vi "ST5 Check Errors.vi"(8 "error in (no error)":errorcluster, 10 "Scan failed":bool, 11 "Read=0":bool) -> (0 "error out":errorcluster)   [LabVIEW 2019]
uses:
  <vilib>/Utility/error.llb/DialogType.ctl
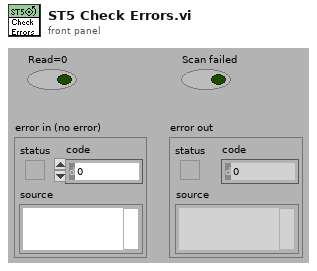
[diagram p1: front panel]
types:
  T1 = typedef "DialogType.ctl" = u16
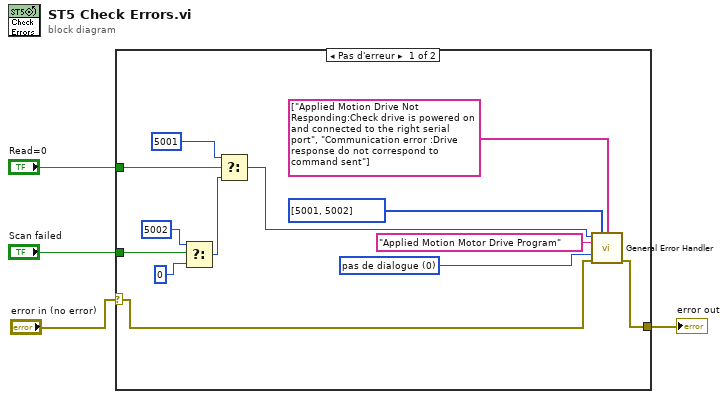
[diagram p0: block diagram]
diagram:
  n1 = case shown="Pas d'erreur" "error in (no error)" {
    selector: "error in (no error)" -> [w5 w18]
    tunnel: "Read=0" -> [w15 _]
    tunnel: "Scan failed" -> [w11 _]
    tunnel: [w6 w18] -> w2
    frame No Error {
      w12 = T1 0 items=["pas de dialogue", "Message OK", "Message continuer ou arrêter", "Message OK + mises en garde", "Arrêter/Continuer + mises en garde"] ("type of dialog (OK msg:1)")
      n2 = Select(t=5002, s=w11, f=0 ("cas faux")) -> (s? t:f=w8:i32)
      n3 = Select(t=5001, s=w15, f=w8) -> (s? t:f=w7:i32)
      n4 = call <vilib>:"General Error Handler.vi"("[error code] (0)"=w7, "[user-defined codes]"=i32[] [5001, 5002], "[user-defined descriptions]"=string[] ["Applied Motion Drive Not Responding:Check drive is powered on and connected to the right serial port", "Communication error :Drive response do not correspond to command sent"], "[error source] (\" \")"="Applied Motion Motor Drive Program" ("[error source] (\" \")"), "type of dialog (OK msg:1)"=w12, "error in (no error)"=w5) -> ("error out"=w6:errorcluster)  [unwired: 5 in, 4 out]
    }
    frame Error {
    }
  }
  "error out" <- w2
